vi "min_max_avg_array (SubVI).vi"(11 "input array":i8[](array[numeric])) -> (1 "min value":i8, 2 "Average":dbl, 3 "max value":i8)   [LabVIEW 2018]
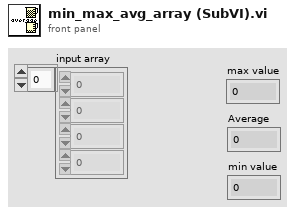
[diagram p1: front panel]
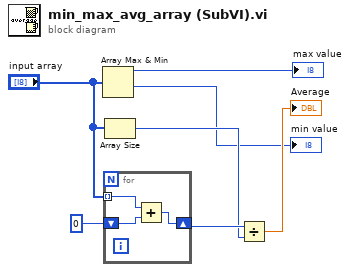
[diagram p0: block diagram]
diagram:
  n1 = Array Max & Min(array="input array") -> (max value=→"max value":i8, min value=→"min value":i8)  [unwired: 2 out]
  n2 = for {
    tunnel: "input array" -> [w9] mode=indexing
    shift-right: [w8] -> w5
    shift-left: i16 0 -> [w10]
    n3 = Add(x=w9, y=w10) -> (x+y=w8:i16)
  }
  n4 = Array Size(array="input array") -> (size(s)=w4:i32)
  n5 = Divide(x=w5, y=w4) -> (x/y=→"Average":dbl)
